vi "Read Analogue.vi"(8 "error in (no error)":errorcluster, 11 "PS in":refnum<class "Sim AI.lvclass">) -> (0 "error out":errorcluster, 2 "Measurements":dbl, 3 "PS out":refnum<class "Sim AI.lvclass">)   [LabVIEW 2019, in "Concrete.lvlib" / "Sim AI.lvclass"]
uses:
  Sim AI.lvclass
  <vilib>/numeric/Random Number (Range) DBL.vi
  Harware Abstraction/Analog In/Analog In.lvclass
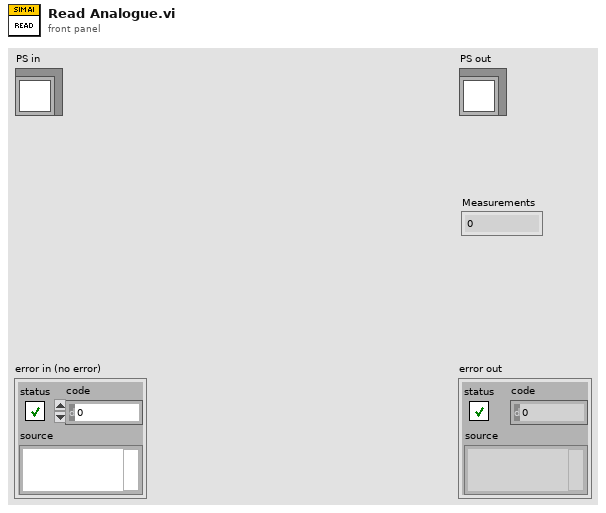
[diagram p1: front panel]
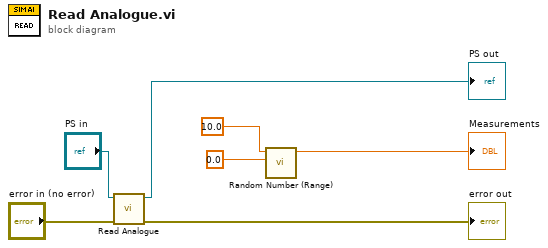
[diagram p0: block diagram]
diagram:
  n1 = call-parent "Read Analogue.vi"("error in (no error)"="error in (no error)", "PS in"="PS in") -> ("error out"=→"error out":errorcluster, "PS out"=→"PS out":refnum<class "Sim AI.lvclass">)  [unwired: 7 in, 1 out]
  n2 = call-poly <vilib>:"Random Number (Range).vi"("lower bound (0)"=0.0, "upper bound (100)"=10.0) -> ("number"=→"Measurements":dbl)  [unwired: 9 in]
